vi "sendcommand.vi"(8 "error in (no error)":errorcluster caption="entrée d'erreur (pas d'erreur)", 11 "para0":string) -> (0 "error out":errorcluster caption="sortie d'erreur", 2 "function return":i32, 3 "para0 out":string)   [LabVIEW 2020, in "Library Instrument & Equipement.lvlib" / "Library Printer.lvlib" / "TSCLIB.lvlib"]
doc: "EXPORT int CALLBACK sendcommand (unsigned char*);"
uses:
  TSCLIB.lvlib
  TSCLIB.dll
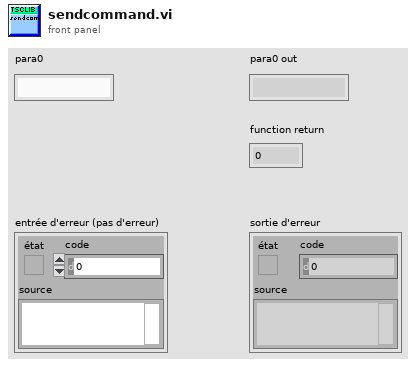
[diagram p1: front panel]
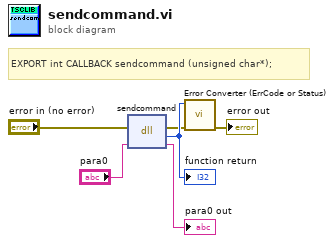
[diagram p0: block diagram]
diagram:
  # "EXPORT int CALLBACK sendcommand (unsigned char*);"
  n1 = dll-call lib="C:/Users/ngarcin/OneDrive - Altyor/Standard TB/Class/Printer/Printer TSC/TSCLIB/TSCLIB.*" fn="sendcommand"(error in="error in (no error)", "para0"="para0") -> (error out=w2:errorcluster, "type de retour"=w6:i32, "para0"=→"para0 out":string)  [unwired: 2 in, 1 out]
  "function return" <- w6
  n2 = call "Error Converter (ErrCode or Status).vi"("error in (no error)"=w2, "error code"=w6) -> ("error out"=→"error out":errorcluster)  [unwired: 9 in]
